vi "Send.vi"(7 "Device Address":u8, 8 "error in (no error)":errorcluster, 9 "eI2Cflags":T1 caption="I2C Flags" items=["None"=0, "START"=2, "REPEATED START"=3, "STOP"=4, "START AND STOP"=6], 10 "Buffer":u8[](array[numeric]), 11 "ProdType_1 in":refnum<class "ProdType_1.lvclass">) -> (0 "error out":errorcluster, 1 "Status":string, 2 "Byte Returned":u32, 3 "ProdType_1 out":refnum<class "ProdType_1.lvclass">)   [LabVIEW 2020, in "I2COUSB.lvlib" / "ProdType_1.lvclass"]
doc: "Send Data"
uses:
  ProdType_1.lvclass
  II2COUSB/II2COUSB/I2CFlags.ctl
  II2COUSB/II2COUSB/II2COUSB.lvclass
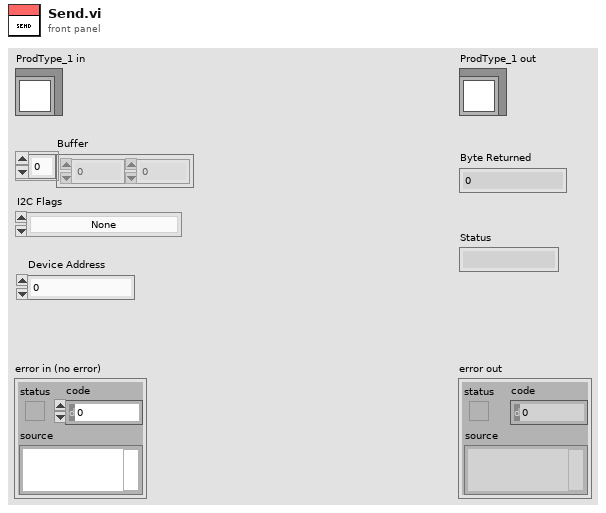
[diagram p1: front panel]
types:
  T1 = typedef "II2COUSB.lvlib/II2COUSB.lvclass/I2CFlags.ctl" = u8
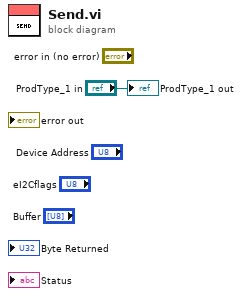
[diagram p0: block diagram]
diagram:
  "ProdType_1 out" <- "ProdType_1 in"
